vi "Start Finite Stream.vi"(8 "error in (no error)":errorcluster, 9 "num samples":u64=1000, 10 "stream index":i32, 11 "refnum in":refnum<k20>) -> (0 "error out":errorcluster, 3 "refnum out":refnum<k20>)   [LabVIEW 2015, in "niInstr Streaming v1 Host.lvlib"]
doc: "Activates the stream to operate in a finite transfer bound by <b>num samples.</b> The stream enters the Finite Transfer state and will autonomously leave the this state in response completing the requested number of samples, or in response to an error state (such as a buffer underflow/overflow condition). A user should monitor the health of the transfer by either using Get Stream State.vi, or through the use of the Wait... functions available in the host API.\n\nWhen a user wishes to prematurely stop a Finite Transfer stream, they should use the appropriate API function to do so. This may be Clear Stream.vi or Stop Stream.vi. Consult the documentation of those VIs for more information.\n\n<B>Input Parameters</B>\n\n<B>error in (no error)</B> 'error in' can accept error information wired from VIs previously called. Use this information to decide if any functionality should be bypassed in the event of errors from other VIs.\n\nRight-click the 'error in' control on the front panel and select 'Explain Error' or 'Explain Warning' from the shortcut menu for more information about the error.\n\n<B>stream index</B> Selects which stream index this VI will interface to. This is the index number at the end of the host interface controls (0..7).\n\n<B>refnum in</B> Wire in the session obtained from Open FPGA Reference.\n\n<B>Output Parameters</B>\n\n<B>error out</B> contains error information. This output provides standard error out functionality.\n\n<B>refnum out</B> Copy of refnum in"
uses:
  <instrlib>/_niInstr/Streaming/v1/Host/niInstr Streaming v1 Host.lvlib
  <instrlib>/_niInstr/Streaming/v1/Host/Public/Stream Host Interface.ctl
  <vilib>/Utility/error.llb/Error Cluster From Error Code.vi
  <vilib>/ErrorRing/Error Ring.xnode
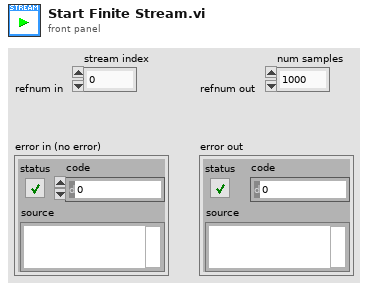
[diagram p1: front panel]
types:
  T1 = typedef "niInstr Streaming v1 Host.lvlib/Stream Host Interface.ctl" = refnum<k20>
  T2 = typedef "niInstr Streaming v1 Common.lvlib/Stream State.ctl" = enum8{"Idle", "Finite Transfer", "Continuous", "Done", "Error", "Not Ready", "Cancel"}
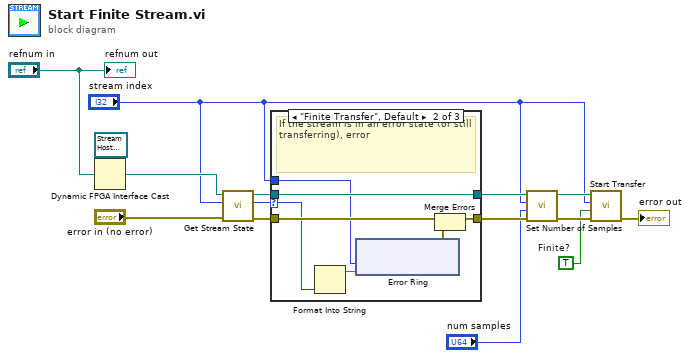
[diagram p0: block diagram]
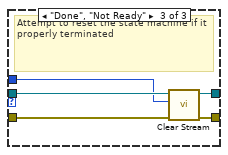
[diagram p3: hidden frame]
diagram:
  w1 = TRUE  # Finite?
  n1 = Dynamic FPGA Interface Cast(Session In=T1 refnum ("Refnum in"), Type="refnum in") -> (Session Out=w8:T1)
  n2 = call <instrlib>:"Get Stream State.vi"("error in (no error)"="error in (no error)", "stream index"="stream index", "refnum in"=w8) -> ("error out"=w11:errorcluster, "stream state"=w12:T2, "refnum out"=w13:T1)  [unwired: 6 in]
  n3 = case shown="\"Finite Transfer\", Default" w12 {
    selector: w12 -> [_ w21 _]
    tunnel: w13 -> [w17 w24 w36]
    tunnel: w11 -> [w16 w23 w37]
    tunnel: "stream index" -> [_ w19 w35]
    tunnel: [w17 w24 w34] -> w9
    tunnel: [w16 w22 w33] -> w10
    frame "Idle" {
      # "If the state machine is already idle, it then it is safe to resume"
    }
    frame "Finite Transfer", Default {
      # "If the stream is in an error state (or still transferring), error"
      n4 = Format Into String(w21) -> (resulting string=w18:string)  [unwired: 3 in, 1 out]
      n5 = xnode "Error Ring"("parameter 0"=w19, "parameter 1"=w18) -> ("error out"=w20:errorcluster)
      n6 = Merge Errors(w23, w20) -> (w22:errorcluster)
    }
    frame "Done", "Not Ready" {
      # "Attempt to reset the state machine if it properly terminated"
      n7 = call <instrlib>:"Clear Stream.vi"("error in (no error)"=w37, "stream index"=w35, "refnum in"=w36) -> ("error out"=w33:errorcluster, "refnum out"=w34:T1)  [unwired: 7 in]
    }
  }
  n8 = call <instrlib>:"Set Number of Samples.vi"("error in (no error)"=w10, "num samples"="num samples", "stream index"="stream index", "refnum in"=w9) -> ("error out"=w5:errorcluster, "refnum out"=w6:T1)  [unwired: 6 in]
  n9 = call <instrlib>:"Start Transfer.vi"("error in (no error)"=w5, "finite?"=w1, "stream index"="stream index", "refnum in"=w6) -> ("error out"=→"error out":errorcluster)  [unwired: 6 in, 1 out]
  "refnum out" <- "refnum in"
